vi "CAlex2_SetLegDH_Squat.vi"(8 "error in (no error)":errorcluster, 9 "End Effector Pos":T1={"Coord4"=[0.0, 0.0, 0.0, 1.0], "ID"=4}, 10 "ArmProperty":T2, 11 "CAlex2 in":refnum<class "CAlex2.lvclass">) -> (0 "error out":errorcluster, 3 "CAlex2 out":refnum<class "CAlex2.lvclass">)   [LabVIEW 2016, in "CAlex2.lvclass"]
uses:
  CAlex2.lvclass
  C:/Users/randh/Desktop/CABLE-LABVIEW/CALEX/CAlex2-controller/Classes/SerialChain/SerialChain.lvclass
  TypeDef/LowerBodyDim.ctl
  SerialChain/TypeDef/PointOnBody.ctl
  SerialChain/TypeDef/xyzO.ctl
  SerialChain/TypeDef/JointType.ctl
  SerialChain/SerialChain.lvclass
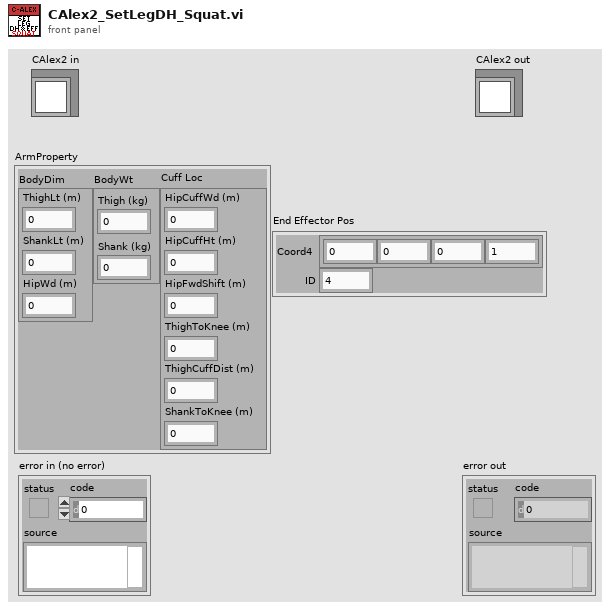
[diagram p1: front panel]
types:
  T1 = typedef "SerialChain.lvclass/PointOnBody.ctl" = cluster{"Coord4":dbl[], "ID":i32}
  T2 = typedef "CAlex2.lvclass/LowerBodyDim.ctl" = cluster{"BodyDim":cluster{"ThighLt (m)":dbl, "ShankLt (m)":dbl, "HipWd (m)":dbl}, "BodyWt":cluster{"Thigh (kg)":dbl, "Shank (kg)":dbl}, "Cuff Loc":cluster{"HipCuffWd (m)":dbl, "HipCuffHt (m)":dbl, "HipFwdShift (m)":dbl, "ThighToKnee (m)":dbl, "ThighCuffDist (m)":dbl, "ShankToKnee (m)":dbl}}
  T3 = typedef "SerialChain.lvclass/JointType.ctl" = enum16{"theta(hinge)", "alpha", "a", "d(slide)"}
  T4 = typedef "SerialChain.lvclass/xyzO.ctl" = enum16{"X", "Y", "Z", "O"}
  T5 = typedef "SerialChain.lvclass/DH_param.ctl" = cluster{"a":dbl, "d":dbl, "theta":dbl, "alpha":dbl, "JointType":T3}
  T6 = cluster{"DH Parameters":T5, "CoM_Pos":T1, "Mass(kg)":dbl}
  T7 = cluster{"DH Parameters":T5, "CoM_Pos":T1, "Mass(kg)":dbl}[]
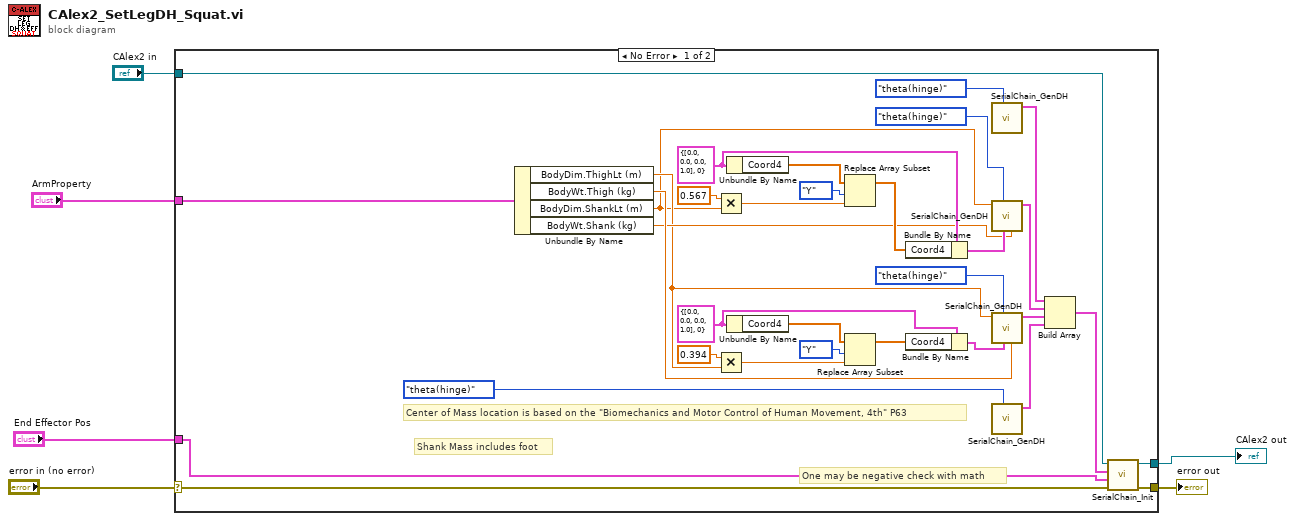
[diagram p0: block diagram]
diagram:
  n1 = case shown="No Error" "error in (no error)" {
    selector: "error in (no error)" -> [w22 w41]
    tunnel: [w15 w41] -> w5
    tunnel: [w14 w40] -> w3
    tunnel: "CAlex2 in" -> [w23 w40]
    tunnel: "ArmProperty" -> [w18 _]
    tunnel: "End Effector Pos" -> [w16 _]
    frame No Error {
      w25 = T1 {"Coord4"=[0.0, 0.0, 0.0, 1.0], "ID"=0} ("CoM_Pos")
      w33 = T1 {"Coord4"=[0.0, 0.0, 0.0, 1.0], "ID"=0} ("CoM_Pos")
      # "One may be negative check with math"
      # "Shank Mass includes foot"
      # "Center of Mass location is based on the \"Biomechanics and Motor Control of Human Movement, 4th\" P63"
      n2 = Unbundle By Name(w18) -> ("BodyDim.ThighLt (m)"=w13:dbl, "BodyWt.Thigh (kg)"=w38:dbl, "BodyDim.ShankLt (m)"=w9:dbl, "BodyWt.Shank (kg)"=w17:dbl)
      n3 = Multiply(x=0.567, y=w9) -> (x*y=w28:dbl)
      n4 = Multiply(x=0.394, y=w13) -> (x*y=w35:dbl)
      n5 = Unbundle By Name(w25) -> ("Coord4"=w29:dbl[])
      n6 = Unbundle By Name(w33) -> ("Coord4"=w34:dbl[])
      n7 = Replace Array Subset(array=w29, new element=w28, index=xyzO."Y" ("XYZ")) -> (w30:dbl[])
      n8 = Replace Array Subset(array=w34, new element=w35, index=xyzO."Y" ("XYZ")) -> (w32:dbl[])
      n9 = Bundle By Name(cluster=w25, "Coord4"=w30) -> (w24:T1)
      n10 = Bundle By Name(cluster=w33, "Coord4"=w32) -> (w31:T1)
      n11 = call "SerialChain_GenDH.vi"("JointType(hinge)"=JointType."theta(hinge)" ("JointType")) -> ("DH Segment Cluster"=w7:T6)  [unwired: 10 in]
      n12 = call "SerialChain_GenDH.vi"("Mass(kg)"=w17, "CoM Position (Origin)"=w24, "JointType(hinge)"=JointType."theta(hinge)" ("JointType"), "a(0)"=w9) -> ("DH Segment Cluster"=w12:T6)  [unwired: 7 in]
      n13 = call "SerialChain_GenDH.vi"("Mass(kg)"=w38, "CoM Position (Origin)"=w31, "JointType(hinge)"=JointType."theta(hinge)" ("JointType"), "a(0)"=w13) -> ("DH Segment Cluster"=w11:T6)  [unwired: 7 in]
      n14 = call "SerialChain_GenDH.vi"("JointType(hinge)"=JointType."theta(hinge)" ("JointType")) -> ("DH Segment Cluster"=w10:T6)  [unwired: 10 in]
      n15 = Build Array(w7, w12, w11, w10) -> (w39:T7)
      n16 = call "SerialChain_Init.vi"("error in (no error)"=w22, "End Effector Pos"=w16, "KnownDHVars"=w39, "SerialChain in"=w23) -> ("error out"=w15:errorcluster, "SerialChain out"=w14:refnum<class "CAlex2.lvclass">)  [unwired: 6 in]
    }
    frame Error {
    }
  }
  "error out" <- w5
  "CAlex2 out" <- w3
